vi "C to F.vi"(11 "celsius":dbl) -> (3 "fahrenheit":dbl)   [LabVIEW 2019, in "Temperature Controller.lvclass"]
uses:
  Temperature Controller.lvclass
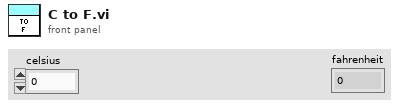
[diagram p1: front panel]
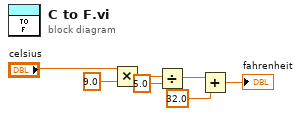
[diagram p0: block diagram]
diagram:
  n1 = Multiply(x="celsius", y=9.0) -> (x*y=w6:dbl)
  n2 = Divide(x=w6, y=5.0) -> (x/y=w4:dbl)
  n3 = Add(x=w4, y=32.0) -> (x+y=→"fahrenheit":dbl)
